vi "Peg-in-hole 2015-03-03 data.vi"() -> ()   [LabVIEW 2013]
uses:
  <vilib>/Analysis/baseanly.llb/Mean (DBL).vi
  <vilib>/Analysis/NI_AALBase.lvlib
  <vilib>/Analysis/NI_AALPro.lvlib
  <vilib>/gmath/NI_Gmath.lvlib
panel:
  in  "y":dbl
  out "correlation coefficient r":dbl
  out "offset":dbl
  out "power":dbl
  out "amplitude":dbl
  out "XY Graph":cluster{cluster{dbl, "mean":dbl}[]}[](graph)
  in  "Times":dbl[](array[numeric])=[35.801, 15.05, 145.25, 25.05, 85.2, 31.05, 196.6, 25.1, 135.5, 25.45, 125.65, 25.3, 55.75, 147.2, 64.85, 25.35, 116.2, 35.45, 85.7, 45.3, 35.3, 15.9, 35.25, 15.45, 65.45, 15.35, 55.35, 14.55, 339.85, 14.65, 86.2, 15.7, 45.45, 15.449, 74.949, 26.0, 68.55, 36.45, 36.2, 26.55, 57.05, 16.65, 25.649, 58.1, 111.0, 25.9, 15.3, 129.8, 55.5, 15.3, 35.3, 15.25, 14.85, 14.55, 35.3, 15.35, 14.95, 15.25, 25.15, 14.6, 14.65, 25.6, 38.05, 15.95, 35.25, 14.75, 35.1, 15.15, 36.05, 15.1, 35.55, 14.85, 25.65, 36.9, 15.1, 14.9, 85.45, 14.5, 37.3, 14.6, 15.3, 15.35, 45.35, 15.25, 65.75, 35.85, 25.25, 15.6, 25.15, 15.35, 15.15, 36.3, 55.95, 15.5, 25.1, 14.5, 96.5, 14.8, 35.2, 14.5, 15.35, 15.65, 15.0, 15.25, 66.8, 15.4, 15.0, 15.35, 15.0, 15.35, 15.3, 15.4, 15.15, 15.35, 14.9, 15.2, 15.05, 15.4, 25.05, 14.65, 14.9, 15.45, 15.2, 15.35, 15.05, 15.45, 55.7, 15.15, 15.05, 15.5, 15.25, 15.65, 46.1, 15.6, 15.0, 15.05, 14.9, 15.4, 14.95, 15.0]
  # "#20-#39 replaced with reruns with peg2\n#40-#56 replaced with reruns with peg3"
  # "Data with one taught point"
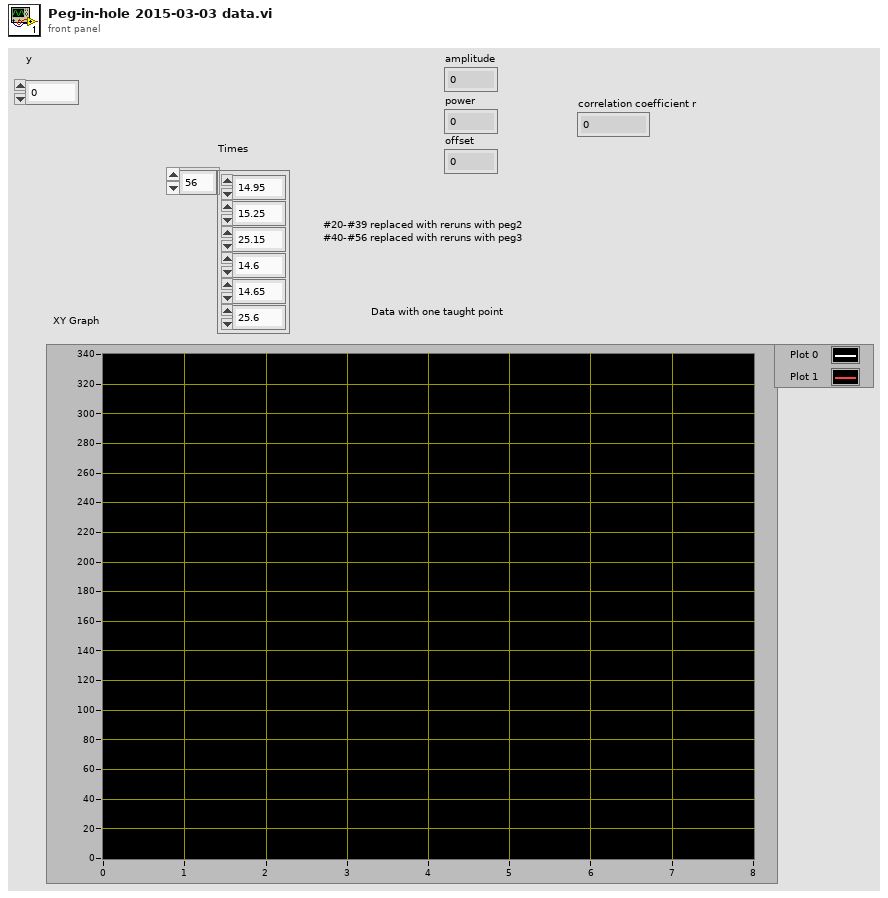
[diagram p1: front panel]
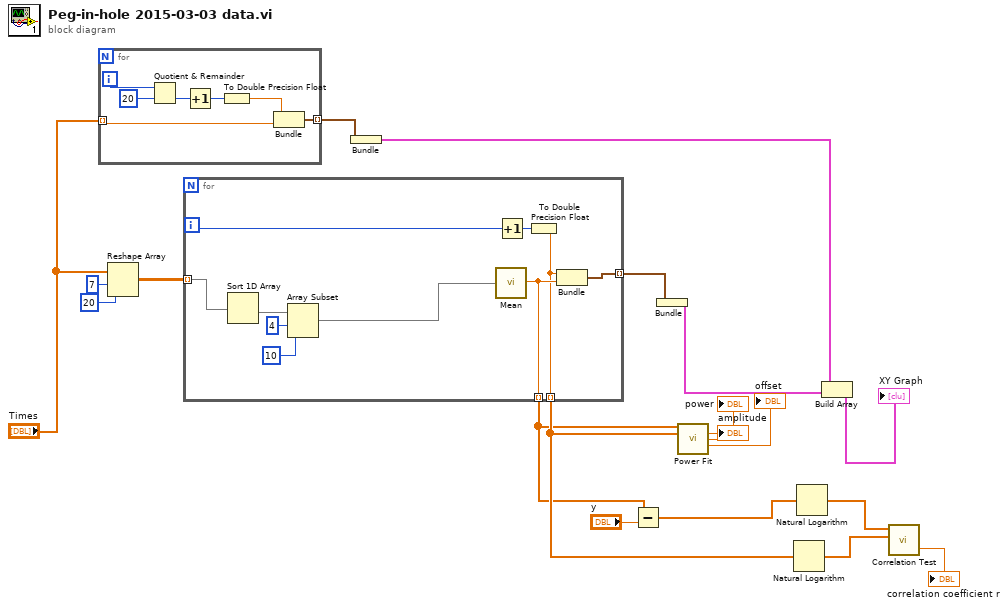
[diagram p0: block diagram]
diagram:
  n1 = for {
    tunnel: "Times" -> [w21] mode=indexing
    tunnel: [w20] -> w14 mode=indexing
    i -> [w26]
    n2 = Quotient & Remainder(x=w26, y=20) -> (floor(x/y)=w24:i32)  [unwired: 1 out]
    n3 = Increment(x=w24) -> (x+1=w23:i32)
    n4 = To Double Precision Float(number=w23) -> (double precision float=w22:dbl)
    n5 = Bundle(w22, w21) -> (w20:cluster{dbl, dbl})  [unwired: 1 in]
  }
  n6 = Reshape Array("Times", 7 ("dimension size"), 20 ("dimension size")) -> (w16:dbl[][])
  n7 = for {
    tunnel: w16 -> [w31] mode=indexing
    tunnel: [w34] -> w15 mode=indexing
    tunnel: [w33] -> w2 mode=indexing
    tunnel: [w32] -> w6 mode=indexing
    i -> [w36]
    n8 = Sort 1D Array(array=w31) -> (sorted array=w30:dbl[])
    n9 = Array Subset(array=w30, index=4, length=10) -> (w27:dbl[])
    n10 = call-poly <vilib>:"Mean.vi"("X"=w27) -> ("mean"=w33:dbl)  [unwired: 1 out]
    n11 = Increment(x=w36) -> (x+1=w35:i32)
    n12 = To Double Precision Float(number=w35) -> (double precision float=w32:dbl)
    n13 = Bundle(w32, "mean"=w33) -> (w34:cluster{dbl, "mean":dbl})  [unwired: 1 in]
  }
  n14 = Bundle(w14) -> (w12:cluster{cluster{dbl, dbl}[]})  [unwired: 1 in]
  n15 = Subtract(x=w2, y="y") -> (x-y=w1:dbl[])
  n16 = Bundle(w15) -> (w11:cluster{cluster{dbl, "mean":dbl}[]})  [unwired: 1 in]
  n17 = call <vilib>:"Power Fit.vi"("Y"=w2, "X"=w6) -> ("amplitude"=→"amplitude":dbl, "power"=→"power":dbl, "offset"=→"offset":dbl)  [unwired: 8 in, 3 out]
  n18 = Natural Logarithm(1:w6) -> (0:w4:dbl[])
  n19 = Natural Logarithm(1:w1) -> (0:w5:dbl[])
  n20 = Build Array(w12, w11) -> (→"XY Graph":cluster{cluster{dbl, "mean":dbl}[]}[])
  n21 = call <vilib>:"Correlation Test.vi"("sample set y"=w4, "sample set x"=w5) -> ("correlation coefficient r"=→"correlation coefficient r":dbl)  [unwired: 5 in, 4 out]
